vi "CRYAuto Save Editor.vi"() -> ()   [LabVIEW 2013]
uses:
  <vilib>/Utility/miscctls.llb/LVBoundsTypeDef.ctl
  Typedef Control/CRYAuto Save Cluster.ctl
  CRYProject/CRYProject Editor Global.vi
  CRYMainGlobal.vi
  CRYWindow/SubVI/CRYMain Sub Window Global.vi
panel:
  out "Auto save Bk":T1 {"Selector" items=["Space", "Underscores", "None"]}
  in  "CurLibChange":bool caption="Add Lib"
  out "EndFlag":bool
  in  "AddStep":bool
  out "Data Names":string[](array[string])
  in  "Board Tab":enum32{"Page 1"}(tab)
  in  "Cancel":bool caption="Apply"
  in  "OK":bool caption="Apply"
  in  "Main Tab":enum32{"Setting", "Help"}(tab)
  in  "Save Op":u16(slide)
  out "Control Mask3 2":bool
  out "Control Mask3":bool
  in  "DBPath":path caption="Select UDL or DSN"
  out "Control Mask2":bool
  out "Control Mask1":bool
  in  "Format Value":bool
  in  "Excel Path":path
  in  "Selector":i32(ring) caption="选择" items=["空格", "下划线", "无"]
  in  "Axes String":string
  in  "User Default":bool caption="使用默认值"
  in  "Custom header":string
  in  "Delimiter":i32(ring) caption="分隔符" items=["制表符", "逗号", "空格", "其他"]
  in  "Autosave Folder Path:":path caption="自动保存文件夹路径"
  out "Save":bool caption="保存"
  in  "Data List":i32[](listbox) caption="数据"
  out "Format":bool caption="格式"
  out "Test Information":bool caption="测试信息"
  in  "Format Op":u16(slide)
  in  "Header Op":u16(slide)
  in  "Add":bool
  in  "Clear":bool
  in  "Template":string caption="模板"
  in  "User defined":string caption="用户定义"
  in  "Operator":bool caption="操作员"
  out "Filename":bool caption="文件名称"
  in  "Character":string caption="字符"
  in  "x":bool
  in  "y":bool
  in  "z":bool
  out "Header":bool caption="标题"
  in  "Layout Op":u16(slide)
  out "Layout":bool caption="布局"
  out "Notation":bool caption="符号"
  in  "Notation Op":u16(slide)
  in  "Notation Decimal":i32 caption="位小数"
  in  "Time":bool caption="时间"
  in  "Lot No.":bool caption="批次"
  in  "Serial No.":bool caption="序号"
  in  "Prompt for comment":bool caption="注释提示"
  in  "File Name Mode1":u16(slide)
  in  "filename constr":i32(listbox)=-1 caption="构造"
  in  "File Name Mode2":u16(slide)
  in  "Axis":u16(slide) caption="轴" scale=0.0..2.0
  in  "Value":u16(ring) caption="曲线库值" items=["Max FSD Out Stimulus", "采集延迟 [Direct In 1]", "unity cal-in sens-in", "CRY33x Mic 1 sens-in", "CRY33x Mic 2 sens-in", "CRY33x Mic 3 sens-in", "CRY33x Mic 4 sens-in", "USB In L sens-in", "USB In R sens-in", "unity cal-out sens-out", "CRY602 Mouth 1 sens-out", "CRY602 Mouth 2 sens-out", "USB Out R sens-out", "Max FSD In [Direct In 1]"]
  out "single val":string
  in  "Help":string
  in  "Apply":bool
  in  "Load...":bool caption="Apply"
  in  "Save As...":bool caption="Apply"
  in  "Revert":bool caption="Apply"
  in  "fn construction":i32[](array[numeric])
  in  "Hardware In":string
  in  "Calibration In":string
  in  "Channel":i32=1
  out "Set up Out":string
  in  "Set up In":string
  in  "stop":bool
  in  "Load Test":bool=TRUE
  out "Auto save":T1 {"Selector" items=["Space", "Underscores", "None"]}
  out "VIMiniumBound":T2
  in  "Proper VI No":i32
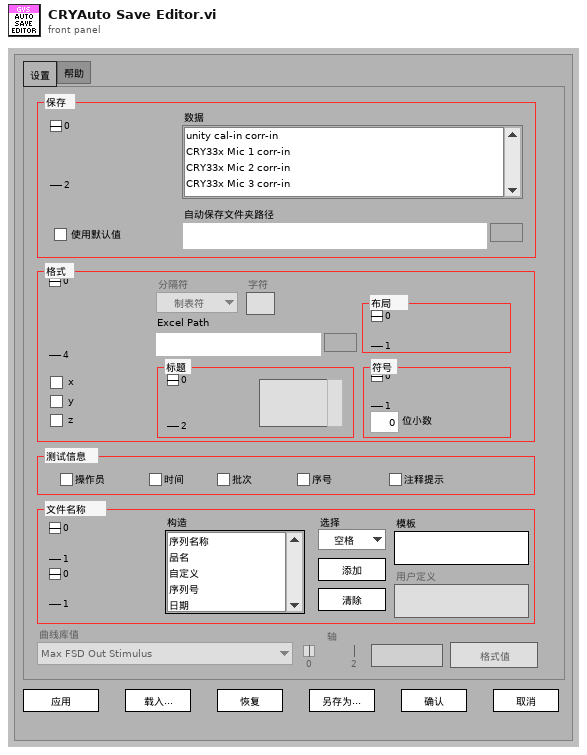
[diagram p1: front panel]
types:
  T1 = typedef "CRYAuto Save Cluster.ctl" = cluster{"Name":string, "save":enum16{"Data", "Results", "Waveforms"}, "Item Names":string[], "Autosave folder":path, "data format":u16, "filename option":enum16{"auto", "prompt"}, "fn construction":i32[], "layout":enum16{"rows", "columns"}, "notation":enum16{"sci", "float"}, "precision":i32, "prompt comment":bool, "header":enum16{"none", "standard", "custom"}, "custom header":string, "serial no.":bool, "User defined":string, "delimiter":enum16{"tab", "comma", "space", "other"}, "other delim":string, "axes":cluster{"x":bool, "y":bool, "z":bool}, "Time Stamp":bool, "Lot No.":bool, "Operator":bool, "Excel Template":string, "New or Append":u16, "Data":u16, "Help":string, "Tab Value":enum32{"Setting", "Help"}, "UDL or DSN":path, "User Default":bool, "Selector":i32, "Axis":u16, "Value Name":string, "format string":cluster{"dB Format String out":string, "Lin Format String out":string}, "DBPath":path}
  T2 = typedef "LVBoundsTypeDef.ctl" = cluster{"Width":u32, "Height":u32}
  T3 = enum32{"existing file", "new file", "new or existing file", "existing dir", "new dir", "new or existing dir", "existing file (use LLBs)", "new file (use LLBs)", "new or existing file (use LLBs)", "new or existing file or directory (use LLBs)", "existing dir (use LLBs)", "new dir (use LLBs)", "new or existing dir (use LLBs)", "existing file or dir", "new file or dir", "new or existing file or dir", "existing file or dir (use LLBs)", "new file or dir (use LLBs)"}
  T4 = typedef "CRYStep.ctl" = cluster{"No.VI":i32, "Category":string, "StepName":string, "Seq setup flattened":string, "Comment":string, "Steps config.":bool[], "Jump config":i32[], "Start":dbl, "Increment":dbl, "Name":string, "Unit":string, "Y data":u16, "Y prefix":string, "Y dB ref":dbl, "Y unit":string, "Repeat State Array":cluster{"Start":dbl, "Increment":dbl, "Count":i32, "Num":i32}[]}
  T5 = enum8{"Enabled", "Disabled", "Disabled and Grayed Out"}
  T6 = enum32{"English", "Chinese", "Korean", "Japanese", "Russian", "Chinese traditional"}
  T7 = enum16{"OK", "Yes", "YesNo", "YesNoCancel", "ReplaceAppend"}
  T8 = typedef "CRYData Cluster Array.ctl" = T9[]
  T9 = typedef "CRYData Cluster.ctl" = cluster{"Name":string, "Curve":cluster{"x":dbl, "y":dbl, "z":dbl}[], "X data":u16, "Y data":u16, "Z data":u16, "X axis":u16, "Y axis":u16, "Z axis":u16, "X unit":string, "Y unit":string, "Z unit":string, "X dB ref":dbl, "Y dB ref":dbl, "Z dB ref":dbl, "single val":bool, "protected":bool, "display X":bool, "display Y":bool, "display Z":bool, "Test Info":string, "Step No.":i32, "Plot Settings":cluster{"Color":u32, "Interpolation":u8, "Point Style":u8, "Line Style":u8, "Point Color":u32, "Line Width":u8, "Bar Plot Style":u8, "Fill To":i16}, "AutoProtect":bool}
  T10 = typedef "CRYResult Cluster Array.ctl" = T11[]
  T11 = typedef "CRYResult Cluster.ctl" = cluster{"Name":string, "Margin":dbl, "unit":string, "Verdict":bool, "Limit":string, "Max/Min":string, "protected":bool, "Step No.":i32, "Test Info":string, "AutoProtect":bool}
  T12 = typedef "CRYWaveform Cluster Array.ctl" = T13[]
  T13 = typedef "CRYWaveform Cluster.ctl" = cluster{"Waveform":cluster{"X0":dbl, "dX":dbl, "Y":sgl[]}, "X data":u16, "Y data":u16, "Y axis":u16, "X unit":string, "Y unit":string, "Y dB ref":dbl, "display Y":bool, "display X":bool, "Overload?":bool, "Test Info":string, "Step No.":i32, "Name":string, "protected":bool, "Sqc history":string[], "Signal Channel ID":i32, "Plot Settings":cluster{"Color":u32, "Interpolation":u8, "Point Style":u8, "Line Style":u8, "Point Color":u32, "Line Width":u8, "Bar Plot Style":u8, "Fill To":i16}, "AutoProtect":bool}
  T14 = cluster{"Apply":bool, "Load Test":bool, "OK":bool, "Cancel":bool}
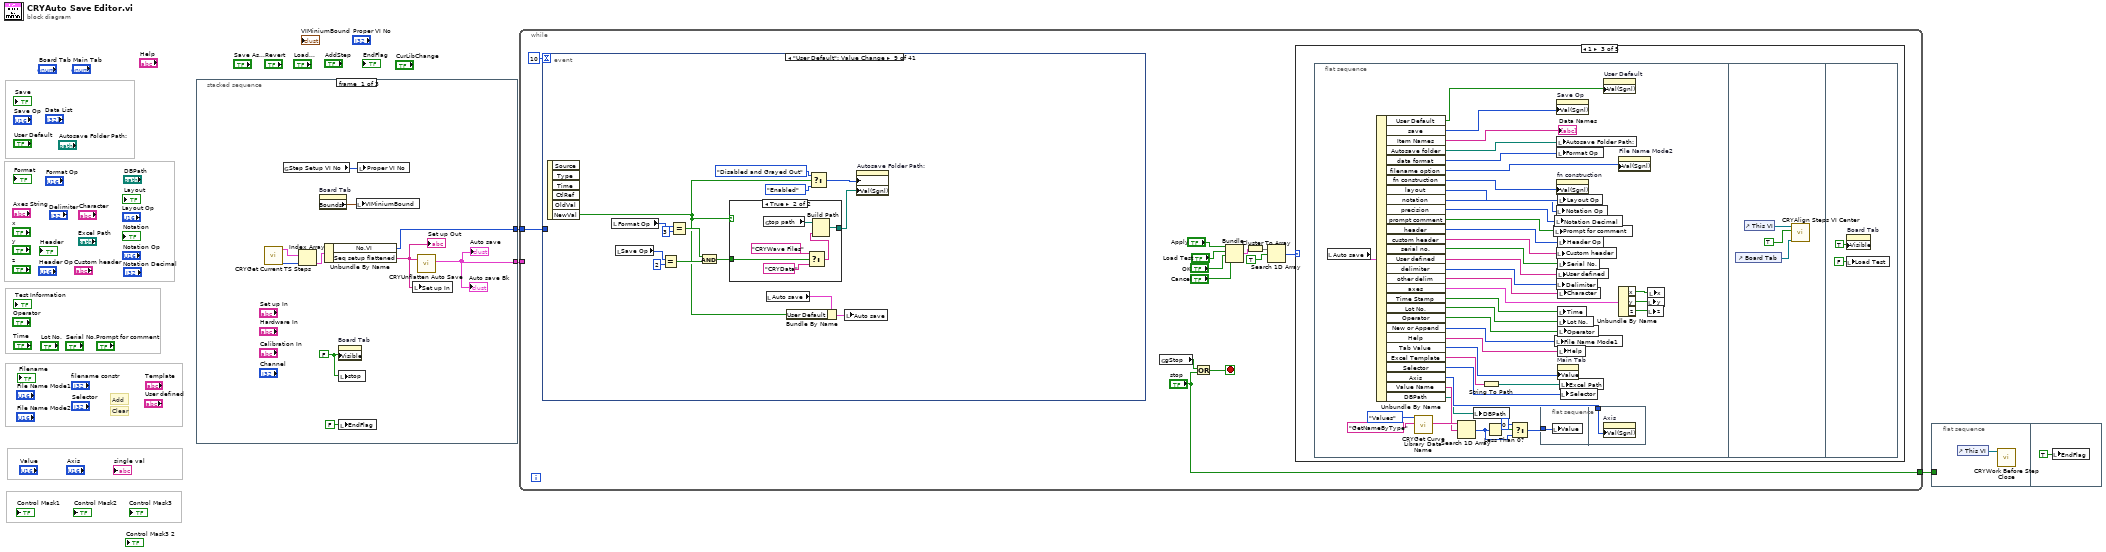
[diagram p0: block diagram]
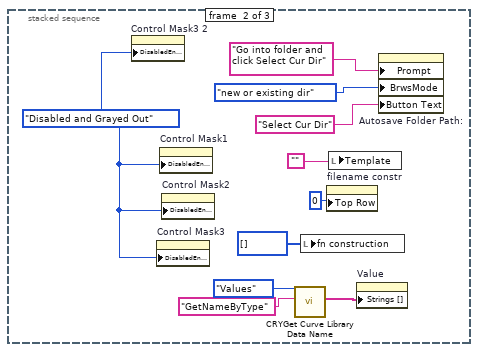
[diagram p2: hidden frame]
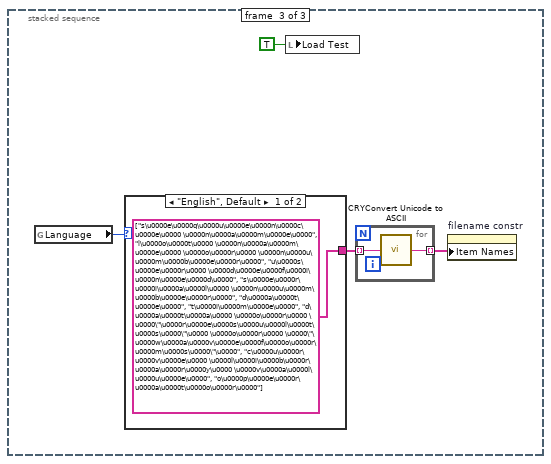
[diagram p3: hidden frame]
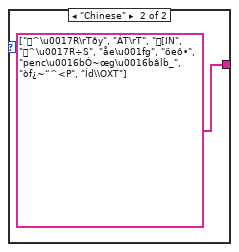
[diagram p4: hidden frame]
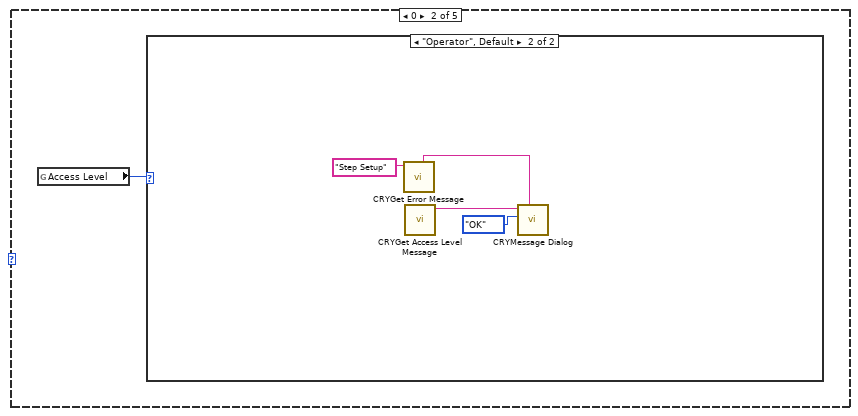
[diagram p6: hidden frame]
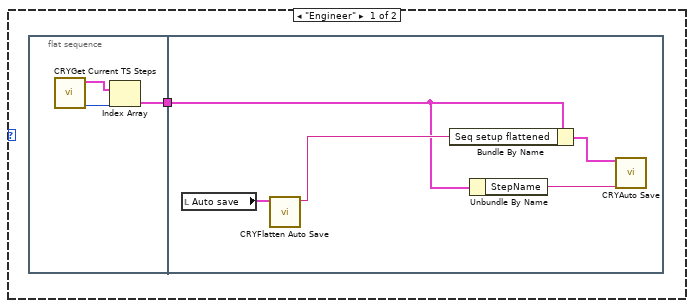
[diagram p7: hidden frame]
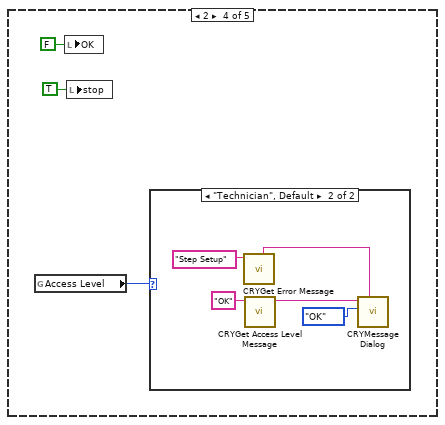
[diagram p8: hidden frame]
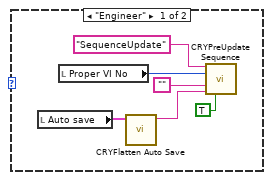
[diagram p9: hidden frame]
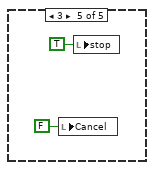
[diagram p10: hidden frame]
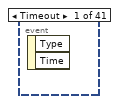
[diagram p11: hidden frame]
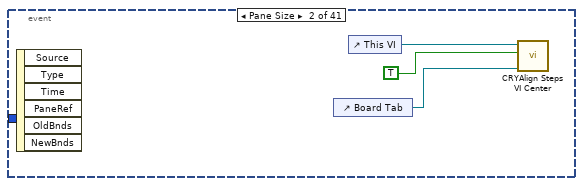
[diagram p12: hidden frame]
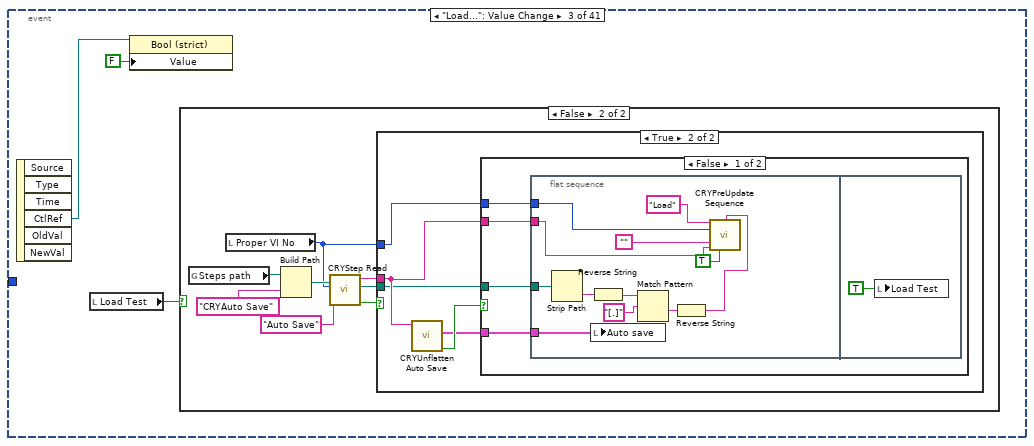
[diagram p13: hidden frame]
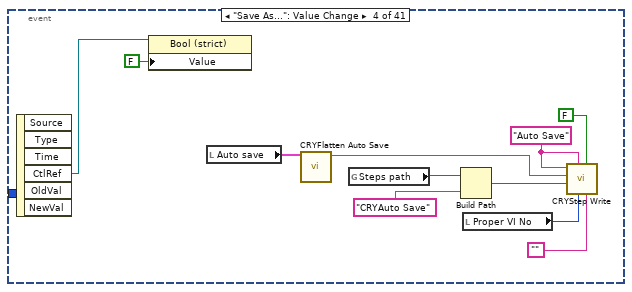
[diagram p17: hidden frame]
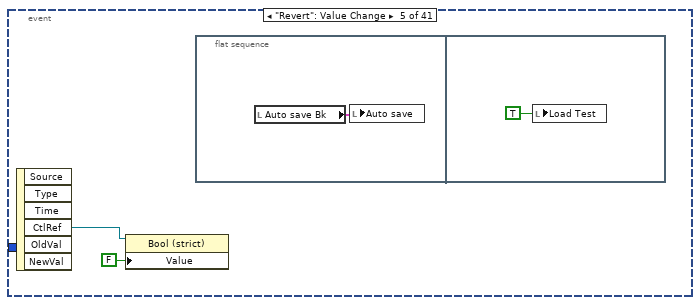
[diagram p18: hidden frame]
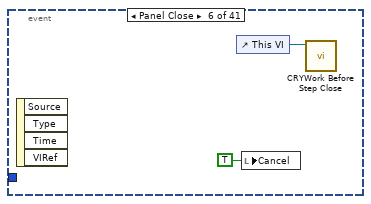
[diagram p19: hidden frame]
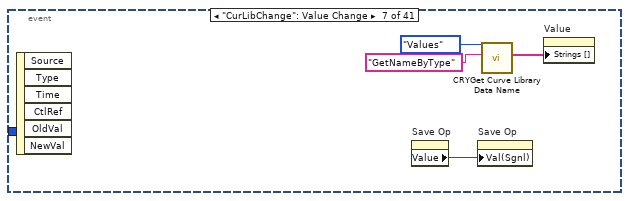
[diagram p20: hidden frame]
diagram:
  # "Clear"
  # "Add"
  n1 = stacked-sequence {
    tunnel: [w5 _ _] -> w3
    tunnel: [w6 _ _] -> w1
    frame #0 {
      w4 = FALSE ("Visible")
      n2 = call "CRYGet Current TS Steps.vi"() -> ("SelectStepNumber in Tree"=w9:i32, "Steps"=w10:T4[])  [unwired: 7 in, 3 out]
      n3 = global read "CRYProject Editor Global.vi" "Step Setup VI No"() -> (w13:i32)
      n4 = Index Array(array=w10, index=w9) -> (element=w12:T4)
      n5 = property on="Board Tab" class="TabCtl (strict)"() -> ("Bounds"=w8:T2)  [unwired: 2 in, 2 out]
      n6 = Unbundle By Name(w12) -> ("No.VI"=w6:i32, "Seq setup flattened"=w11:string)
      "Set up Out" <- w11
      n7 = property on="Board Tab" class="TabCtl (strict)"("Visible"=w4) -> ()  [unwired: 2 in, 2 out]
      n8 = local write "stop"(w4) -> ()
      n9 = local write "EndFlag"(FALSE ("EndFlag")) -> ()
      n10 = local write "VIMiniumBound"(w8) -> ()
      n11 = local write "Proper VI No"(w13) -> ()
      n12 = local write "Set up In"(w11) -> ()
      n13 = call "CRYUnflatten Auto Save.vi"("Flatten Auto Save"=w11) -> ("Auto save"=w5:T1)  [unwired: 8 in, 2 out]
      "Auto save" <- w5
      "Auto save Bk" <- w5
    }
    frame #1 {
      w14 = T5."Disabled and Grayed Out" ("Disabled")
      n14 = property on="Control Mask3 2" class="Bool (strict)"("DisabledEnum"=w14) -> ()  [unwired: 2 in, 2 out]
      n15 = property on="Control Mask3" class="Bool (strict)"("DisabledEnum"=w14) -> ()  [unwired: 2 in, 2 out]
      n16 = property on="Control Mask1" class="Bool (strict)"("DisabledEnum"=w14) -> ()  [unwired: 2 in, 2 out]
      n17 = property on="Control Mask2" class="Bool (strict)"("DisabledEnum"=w14) -> ()  [unwired: 2 in, 2 out]
      n18 = call "CRYGet Curve Library Data Name.vi"("sAction"="GetNameByType", "Type"=enum16{"Curves", "Values", "Results", "WFM"}."Values") -> ("sNames"=w16:string[])  [unwired: 6 in, 3 out]
      n19 = local write "fn construction"(i32[] [] ("fn construction")) -> ()
      n20 = property on="filename constr" class="LstBox (strict)"("Top Row"=0 ("filename constr")) -> ()  [unwired: 2 in, 2 out]
      n21 = local write "Template"("") -> ()
      n22 = property on="Value" class="Ring (strict)"("Strings []"=w16) -> ()  [unwired: 2 in, 2 out]
      n23 = property on="Autosave Folder Path:" class="Path"("Prompt"="Go into folder and click Select Cur Dir" ("prompt"), "BrwsMode"=T3."new or existing dir" ("Browse Options:Selection Mode"), "Button Text"="Select Cur Dir" ("Browse Options:Button Text")) -> ()  [unwired: 2 in, 2 out]
    }
    frame #2 {
      n24 = global read "CRYMainGlobal.vi" "Language"() -> (w26:T6)
      n25 = case shown="\"English\", Default" w26 {
        tunnel: [string[] ["s\u0000e\u0000q\u0000u\u0000e\u0000n\u0000c\u0000e\u0000 \u0000n\u0000a\u0000m\u0000e\u0000", "l\u0000o\u0000t\u0000 \u0000n\u0000a\u0000m\u0000e\u0000 \u0000o\u0000r\u0000 \u0000n\u0000u\u0000m\u0000b\u0000e\u0000r\u0000", "u\u0000s\u0000e\u0000r\u0000 \u0000d\u0000e\u0000f\u0000i\u0000n\u0000e\u0000d\u0000", "s\u0000e\u0000r\u0000i\u0000a\u0000l\u0000 \u0000n\u0000u\u0000m\u0000b\u0000e\u0000r\u0000", "d\u0000a\u0000t\u0000e\u0000", "t\u0000i\u0000m\u0000e\u0000", "d\u0000a\u0000t\u0000a\u0000 \u0000o\u0000r\u0000 \u0000\"\u0000r\u0000e\u0000s\u0000u\u0000l\u0000t\u0000s\u0000\"\u0000 \u0000o\u0000r\u0000 \u0000\"\u0000w\u0000a\u0000v\u0000e\u0000f\u0000o\u0000r\u0000m\u0000s\u0000\"\u0000", "c\u0000u\u0000r\u0000v\u0000e\u0000 \u0000l\u0000i\u0000b\u0000r\u0000a\u0000r\u0000y\u0000 \u0000v\u0000a\u0000l\u0000u\u0000e\u0000", "o\u0000p\u0000e\u0000r\u0000a\u0000t\u0000o\u0000r\u0000"] string[] ["^\u0017R\rTðy", "ÁT\rT", "ꁚ[IN", "^\u0017R÷S", "åe\u001fg", "öeô•", "penc\u0016bÓ~œg\u0016bâlb_", "òf¿~“^<P", "Íd\\OXT"]] -> w25
        frame "English", Default {
        }
        frame "Chinese" {
        }
      }
      n26 = local write "Load Test"(TRUE ("Load Test")) -> ()
      n27 = for {
        tunnel: [w31] -> w24 mode=indexing
        tunnel: w25 -> [w30] mode=indexing
        n28 = call "CRYConvert Unicode to ASCII.vi"("Unicode"=w30) -> ("ASCII"=w31:string)  [unwired: 4 in]
      }
      n29 = property on="filename constr" class="LstBox (strict)"("Item Names"=w24) -> ()  [unwired: 2 in, 2 out]
    }
  }
  n30 = while {
    tunnel: w3 -> [_]
    tunnel: ["stop"] -> w2
    tunnel: w1 -> [w35]
    stop <- w38 stop-if-true
    n31 = event shown="[8] \"User Default\": Value Change" {
      selector: _ -> [_ _ _ _ _ _ _ _ _ _ _ _ _ _ _ _ _ _ _ _ _ _ _ _ _ _ _ _ _ _ _ _ _ _ _ _ _ _ _ _ _]
      dyn-events: _ -> [_ _ _ _ _ _ _ _ _ _ _ _ _ _ _ _ _ _ _ _ _ _ _ _ _ _ _ _ _ _ _ _ _ _ _ _ _ _ _ _ _]
      timeout: 10 -> [_ _ _ _ _ _ _ _ _ _ _ _ _ _ _ _ _ _ _ _ _ _ _ _ _ _ _ _ _ _ _ _ _ _ _ _ _ _ _ _ _]
      tunnel: w35 -> [_ _ _ _ _ _ _ w183 _ _ _ _ _ _ _ _ _ _ _ _ _ _ _ _ _ _ _ _ _ _ _ _ _ _ _ _ _ _ _ _ _]
      event Timeout {
        n32 = event-data() -> ()  [unwired: 3 out]
      }
      event Pane Size {
        n33 = event-data() -> ()  [unwired: 7 out]
        n34 = control-ref of="Board Tab"() -> (w124:refnum<vi>)
        n35 = control-ref of="This VI"() -> (w123:refnum<vi>)
        n36 = call "CRYAlign Steps VI Center.vi"("Tab2"=w124, "Input/Output"=TRUE ("Preview"), "VIRef"=w123) -> ()  [unwired: 1 in, 8 out]
      }
      event "Load...": Value Change {
        n37 = event-data() -> ("CtlRef"=w126:refnum<vi>)  [unwired: 6 out]
        n38 = local read "Load Test"() -> (w128:bool)
        n39 = property class="Bool (strict)"(reference=w126, "Value"=FALSE) -> ()  [unwired: 1 in, 2 out]
        n40 = case shown="False" w128 {
          frame True {
          }
          frame False {
            n41 = global read "CRYMainGlobal.vi" "Steps path"() -> (w135:path)
            n42 = local read "Proper VI No"() -> (w130:i32)
            n43 = Build Path(base path=w135, name or relative path="CRYAuto Save") -> (appended path=w134:path)
            n44 = call "CRYStep Read.vi"("Category Name"="Auto Save", "Proper VI No"=w130, "Step File Path"=w134) -> ("status"=w132:bool, "selected path"=w129:path, "Flatten Step"=w131:string)  [unwired: 1 in, 3 out]
            n45 = case shown="True" w132 {
              tunnel: w131 -> [_ w138]
              tunnel: w130 -> [_ w139]
              tunnel: w129 -> [_ w137]
              frame False {
              }
              frame True {
                n46 = call "CRYUnflatten Auto Save.vi"("Flatten Auto Save"=w138) -> ("Error?"=w141:bool, "Auto save"=w140:T1)  [unwired: 8 in, 1 out]
                n47 = case shown="False" w141 {
                  tunnel: w140 -> [w145 _]
                  tunnel: w139 -> [w144 _]
                  tunnel: w138 -> [w143 _]
                  tunnel: w137 -> [w142 _]
                  frame False {
                    n48 = flat-sequence {
                      tunnel: w145 -> [w157]
                      tunnel: w144 -> [w154]
                      tunnel: w143 -> [w153]
                      tunnel: w142 -> [w152]
                      frame #0 {
                        n49 = Strip Path(path=w152) -> (name=w147:string)  [unwired: 1 out]
                        n50 = local write "Auto save"(w157) -> ()
                        n51 = Reverse String(1:w147) -> (0:w149:string)
                        n52 = Match Pattern(string=w149, regular expression="[.]") -> (after substring=w150:string)  [unwired: 4 out]
                        n53 = Reverse String(1:w150) -> (0:w146:string)
                        n54 = call "CRYPreUpdate Sequence.vi"("EventName"="Load", "StepName Arg3"=w146, "Proper VI No"=w154, "Project View Step Name Identifier Arg1"="", "Step flattened Arg2"=w153, "AllChangeFlg"=TRUE ("Name/Identifier")) -> ()  [unwired: 10 in]
                      }
                      frame #1 {
                        n55 = local write "Load Test"(TRUE ("Load Test")) -> ()
                      }
                    }
                  }
                  frame True {
                  }
                }
              }
            }
          }
        }
      }
      event "Save As...": Value Change {
        w163 = "Auto Save" ("Step File Name")
        n56 = event-data() -> ("CtlRef"=w159:refnum<vi>)  [unwired: 6 out]
        n57 = property class="Bool (strict)"(reference=w159, "Value"=FALSE) -> ()  [unwired: 1 in, 2 out]
        n58 = local read "Auto save"() -> (w161:T1)
        n59 = call "CRYFlatten Auto Save.vi"("Auto Save"=w161) -> ("Auto Save flattened"=w162:string)  [unwired: 10 in]
        n60 = global read "CRYMainGlobal.vi" "Steps path"() -> (w165:path)
        n61 = Build Path(base path=w165, name or relative path="CRYAuto Save") -> (appended path=w164:path)
        n62 = local read "Proper VI No"() -> (w168:i32)
        n63 = call "CRYStep Write.vi"("StepIdentifier"="", "Default"=FALSE, "Proper VI No"=w168, "Category Name"=w163, "Step File Path"=w164, "Step flattened"=w162, "Step File Name"=w163) -> ()  [unwired: 1 in, 4 out]
      }
      event "Revert": Value Change {
        n64 = event-data() -> ("CtlRef"=w171:refnum<vi>)  [unwired: 6 out]
        n65 = property class="Bool (strict)"(reference=w171, "Value"=FALSE) -> ()  [unwired: 1 in, 2 out]
        n66 = flat-sequence {
          frame #0 {
            n67 = local read "Auto save Bk"() -> (w172:T1)
            n68 = local write "Auto save"(w172) -> ()
          }
          frame #1 {
            n69 = local write "Load Test"(TRUE ("Load Test")) -> ()
          }
        }
      }
      event Panel Close {
        n70 = event-data() -> ()  [unwired: 5 out]
        n71 = control-ref of="This VI"() -> (w175:refnum<vi>)
        n72 = local write "Cancel"(TRUE ("Cancel")) -> ()
        n73 = call "CRYWork Before Step Close.vi"("StepVI Ref"=w175) -> ()  [unwired: 11 in]
      }
      event "CurLibChange": Value Change {
        n74 = event-data() -> ()  [unwired: 7 out]
        n75 = property on="Save Op" class="Slide (strict)"() -> ("Value"=w176:u16)  [unwired: 2 in, 2 out]
        n76 = property on="Save Op" class="Slide (strict)"("Val(Sgnl)"=w176) -> ()  [unwired: 2 in, 2 out]
        n77 = call "CRYGet Curve Library Data Name.vi"("sAction"="GetNameByType", "Type"=enum16{"Curves", "Values", "Results", "WFM"}."Values") -> ("sNames"=w179:string[])  [unwired: 6 in, 3 out]
        n78 = property on="Value" class="Ring (strict)"("Strings []"=w179) -> ()  [unwired: 2 in, 2 out]
      }
      event "Save Op": Value Change {
        n79 = event-data() -> ("NewVal"=w189:u16)  [unwired: 6 out]
        n80 = global read "CRYMainGlobal.vi" "On/Off Line"() -> (w187:bool)
        n81 = call "CRYGet Error Message.vi"("Kind"="Auto Save Sub") -> ("Unicode Message Sub"=w185:string[])  [unwired: 5 in, 5 out]
        n82 = for {
          tunnel: w185 -> [w197] mode=indexing
          tunnel: [w196] -> w184 mode=indexing
          n83 = call "CRYConvert Unicode to ASCII.vi"("Unicode"=w197) -> ("ASCII"=w196:string)  [unwired: 4 in]
        }
        n84 = Index Array(array=w184, index=w189) -> (element=w188:string)
        n85 = case shown="2" w189 {
          tunnel: w183 -> [w206 w231 w246]
          tunnel: [w205 w230 w245] -> w193
          tunnel: [enum16{"Data", "Results", "Waveforms"}."Data" ("save") enum16{"Data", "Results", "Waveforms"}."Results" ("save") enum16{"Data", "Results", "Waveforms"}."Waveforms" ("save")] -> w191
          tunnel: w188 -> [w203 w228 w243]
          tunnel: w187 -> [w202 w227 w242]
          tunnel: [w201 w226 w241] -> w182
          frame 0, Default {
            n86 = case shown="True" w202 {
              tunnel: enum16{"Curves", "Values", "Results", "WFM"}."Curves" ("Type In") -> [w215 w221]
              tunnel: enum16{"Curves", "Values", "Results", "WFM"}."Values" ("Type In") -> [w216 w220]
              tunnel: [w214 w219] -> w210
              tunnel: [w213 w218] -> w209
              tunnel: w206 -> [_ w217]
              frame False {
                n87 = call "CRYGet Curve Library Array.vi"("Type In"=w215) -> ("Curve/Value array"=w214:T8)  [unwired: 10 out]
                n88 = call "CRYGet Curve Library Array.vi"("Type In"=w216) -> ("Curve/Value array"=w213:T8)  [unwired: 10 out]
              }
              frame True {
                n89 = call "CRYGet Upper Step Data.vi"("Type In"=w221, "No.VI"=w217) -> ("Curve array"=w219:T8)  [unwired: 9 out]
                n90 = call "CRYGet Upper Step Data.vi"("Type In"=w220, "No.VI"=w217) -> ("Value array"=w218:T8)  [unwired: 9 out]
              }
            }
            n91 = for {
              tunnel: w210 -> [w225] mode=indexing
              tunnel: [w224] -> w208 mode=indexing
              n92 = Unbundle By Name(w225) -> ("Name"=w224:string)
            }
            n93 = for {
              tunnel: w209 -> [w223] mode=indexing
              tunnel: [w222] -> w207 mode=indexing
              n94 = Unbundle By Name(w223) -> ("Name"=w222:string)
            }
            n95 = Build Array (concatenate)(w208, w207) -> (w205:string[])
            n96 = property on="Data List" class="LstBox (strict)"("Item Names"=w205, "Caption.Text"=w203) -> (error out=w201:errorcluster)  [unwired: 2 in, 1 out]
          }
          frame 1 {
            n97 = case shown="True" w227 {
              tunnel: enum16{"Curves", "Values", "Results", "WFM"}."Results" ("Type In") -> [w235 w238]
              tunnel: [w234 w237] -> w232
              tunnel: w231 -> [_ w236]
              frame False {
                n98 = call "CRYGet Curve Library Array.vi"("Type In"=w235) -> ("Result array"=w234:T10)  [unwired: 10 out]
              }
              frame True {
                n99 = call "CRYGet Upper Step Data.vi"("Type In"=w238, "No.VI"=w236) -> ("Result array"=w237:T10)  [unwired: 9 out]
              }
            }
            n100 = for {
              tunnel: w232 -> [w240] mode=indexing
              tunnel: [w239] -> w230 mode=indexing
              n101 = Unbundle By Name(w240) -> ("Name"=w239:string)
            }
            n102 = property on="Data List" class="LstBox (strict)"("Item Names"=w230, "Caption.Text"=w228) -> (error out=w226:errorcluster)  [unwired: 2 in, 1 out]
          }
          frame 2 {
            n103 = case shown="True" w242 {
              tunnel: enum16{"Curves", "Values", "Results", "WFM"}."WFM" ("Type In") -> [w250 w253]
              tunnel: [w249 w252] -> w247
              tunnel: w246 -> [_ w251]
              frame False {
                n104 = call "CRYGet Curve Library Array.vi"("Type In"=w250) -> ("Waveform Array"=w249:T12)  [unwired: 10 out]
              }
              frame True {
                n105 = call "CRYGet Upper Step Data.vi"("Type In"=w253, "No.VI"=w251) -> ("Waveform Array"=w252:T12)  [unwired: 9 out]
              }
            }
            n106 = for {
              tunnel: w247 -> [w255] mode=indexing
              tunnel: [w254] -> w245 mode=indexing
              n107 = Unbundle By Name(w255) -> ("Name"=w254:string)
            }
            n108 = property on="Data List" class="LstBox (strict)"("Item Names"=w245, "Caption.Text"=w243) -> (error out=w241:errorcluster)  [unwired: 2 in, 1 out]
          }
        }
        n109 = local read "Data Names"() -> (w192:string[])
        n110 = local read "Auto save"() -> (w194:T1)
        n111 = local read "Format Op"() -> (w195:u16)
        n112 = Bundle By Name(cluster=w194, "save"=w191) -> (w186:T1)
        n113 = for {
          tunnel: w193 -> [w199]
          tunnel: w192 -> [w200] mode=indexing
          tunnel: [w198] -> w181 mode=indexing
          n114 = Search 1D Array(1D array=w199, element=w200) -> (index of element=w198:i32)  [unwired: 1 in]
        }
        n115 = property on="Data List" class="LstBox (strict)"(error in=w182, "Top Row"=0) -> ()  [unwired: 1 in, 2 out]
        n116 = local write "Auto save"(w186) -> ()
        n117 = property on="Format Op" class="Slide (strict)"("Val(Sgnl)"=w195) -> ()  [unwired: 2 in, 2 out]
        n118 = local write "Data List"(w181) -> ()
      }
      event "User Default": Value Change {
        n119 = event-data() -> ("NewVal"=w257:bool)  [unwired: 6 out]
        n120 = local read "Format Op"() -> (w264:u16)
        n121 = local read "Save Op"() -> (w261:u16)
        n122 = Equal?(x=w261, y=u16 2) -> (x = y?=w259:bool)
        n123 = Equal?(x=w264, y=u16 3) -> (x = y?=w260:bool)
        n124 = And(x=w260, y=w259) -> (x .and. y?=w258:bool)
        n125 = case shown="True" w257 {
          tunnel: [w270 w274] -> w263
          tunnel: w258 -> [_ w276]
          frame False {
            n126 = local read "Autosave Folder Path:"() -> (w270:path)
          }
          frame True {
            n127 = global read "CRYMainGlobal.vi" "top path"() -> (w275:path)
            n128 = Select(t="CRYWave Files", s=w276, f="CRYData") -> (s? t:f=w271:string)
            n129 = Build Path(base path=w275, name or relative path=w271) -> (appended path=w274:path)
          }
        }
        n130 = local read "Auto save"() -> (w269:T1)
        n131 = Bundle By Name(cluster=w269, "User Default"=w257) -> (w268:T1)
        n132 = Select(t=T5."Disabled and Grayed Out" ("Disabled"), s=w257, f=T5."Enabled" ("Disabled")) -> (s? t:f=w256:T5)
        n133 = local write "Auto save"(w268) -> ()
        n134 = property on="Autosave Folder Path:" class="Path"("DisabledEnum"=w256, "Val(Sgnl)"=w263) -> ()  [unwired: 2 in, 2 out]
      }
      event "Format Op": Value Change {
        n135 = event-data() -> ("NewVal"=w278:u16)  [unwired: 6 out]
        n136 = case shown="4" w278 {
          frame 0, Default {
            w281 = TRUE ("Visible")
            w280 = FALSE ("Visible")
            w283 = T5."Enabled" ("Disabled")
            # "Text"
            n137 = property on="x" class="Bool (strict)"("DisabledEnum"=w283) -> ()  [unwired: 2 in, 2 out]
            n138 = property on="Delimiter" class="Ring (strict)"("DisabledEnum"=w283) -> ()  [unwired: 2 in, 2 out]
            n139 = property on="Notation Decimal" class="DigNum (strict)"("DisabledEnum"=w283) -> ()  [unwired: 2 in, 2 out]
            n140 = property on="Operator" class="Bool (strict)"("DisabledEnum"=w283) -> ()  [unwired: 2 in, 2 out]
            n141 = property on="Prompt for comment" class="Bool (strict)"("DisabledEnum"=w283) -> ()  [unwired: 2 in, 2 out]
            n142 = property on="Excel Path" class="Path"("DisabledEnum"=T5."Disabled and Grayed Out" ("Disabled")) -> ()  [unwired: 2 in, 2 out]
            n143 = property on="y" class="Bool (strict)"("DisabledEnum"=w283) -> ()  [unwired: 2 in, 2 out]
            n144 = property on="Layout Op" class="Slide (strict)"("DisabledEnum"=w283) -> ()  [unwired: 2 in, 2 out]
            n145 = property on="Time" class="Bool (strict)"("DisabledEnum"=w283) -> ()  [unwired: 2 in, 2 out]
            n146 = property on="Header Op" class="Slide (strict)"("DisabledEnum"=w283) -> ()  [unwired: 2 in, 2 out]
            n147 = property on="z" class="Bool (strict)"("DisabledEnum"=w283) -> ()  [unwired: 2 in, 2 out]
            n148 = property on="Notation Op" class="Slide (strict)"("DisabledEnum"=w283) -> ()  [unwired: 2 in, 2 out]
            n149 = property on="Lot No." class="Bool (strict)"("DisabledEnum"=w283) -> ()  [unwired: 2 in, 2 out]
            n150 = property on="Serial No." class="Bool (strict)"("DisabledEnum"=w283) -> ()  [unwired: 2 in, 2 out]
            n151 = local read "Header Op"() -> (w284:u16)
            n152 = local read "Delimiter"() -> (w285:i32)
            n153 = property on="Delimiter" class="Ring (strict)"("Val(Sgnl)"=w285) -> ()  [unwired: 2 in, 2 out]
            n154 = property on="Header Op" class="Slide (strict)"("Val(Sgnl)"=w284) -> ()  [unwired: 2 in, 2 out]
            n155 = property on="Control Mask1" class="Bool (strict)"("Visible"=w280) -> ()  [unwired: 2 in, 2 out]
            n156 = property on="Control Mask2" class="Bool (strict)"("Visible"=w280) -> ()  [unwired: 2 in, 2 out]
            n157 = property on="DBPath" class="Path"("Visible"=w280) -> ()  [unwired: 2 in, 2 out]
            n158 = property on="Control Mask3" class="Bool (strict)"("Visible"=w280) -> ()  [unwired: 2 in, 2 out]
            n159 = property on="Layout" class="Bool (strict)"("Visible"=w281) -> ()  [unwired: 2 in, 2 out]
            n160 = property on="Layout Op" class="Slide (strict)"("Visible"=w281) -> ()  [unwired: 2 in, 2 out]
          }
          frame 1 {
            w287 = TRUE ("Visible")
            w286 = FALSE ("Visible")
            w289 = T5."Enabled" ("Disabled")
            w288 = T5."Disabled and Grayed Out" ("Disabled")
            # "DAT/RES/WFM"
            # "Result"
            n161 = property on="Operator" class="Bool (strict)"("DisabledEnum"=w289) -> ()  [unwired: 2 in, 2 out]
            n162 = property on="Prompt for comment" class="Bool (strict)"("DisabledEnum"=w289) -> ()  [unwired: 2 in, 2 out]
            n163 = property on="Time" class="Bool (strict)"("DisabledEnum"=w289) -> ()  [unwired: 2 in, 2 out]
            n164 = property on="x" class="Bool (strict)"("DisabledEnum"=w288) -> ()  [unwired: 2 in, 2 out]
            n165 = property on="Delimiter" class="Ring (strict)"("DisabledEnum"=w288) -> ()  [unwired: 2 in, 2 out]
            n166 = property on="Notation Decimal" class="DigNum (strict)"("DisabledEnum"=w288) -> ()  [unwired: 2 in, 2 out]
            n167 = property on="Lot No." class="Bool (strict)"("DisabledEnum"=w289) -> ()  [unwired: 2 in, 2 out]
            n168 = property on="y" class="Bool (strict)"("DisabledEnum"=w288) -> ()  [unwired: 2 in, 2 out]
            n169 = property on="Layout Op" class="Slide (strict)"("DisabledEnum"=w288) -> ()  [unwired: 2 in, 2 out]
            n170 = property on="Header Op" class="Slide (strict)"("DisabledEnum"=w288) -> ()  [unwired: 2 in, 2 out]
            n171 = property on="Serial No." class="Bool (strict)"("DisabledEnum"=w289) -> ()  [unwired: 2 in, 2 out]
            n172 = property on="z" class="Bool (strict)"("DisabledEnum"=w288) -> ()  [unwired: 2 in, 2 out]
            n173 = property on="Notation Op" class="Slide (strict)"("DisabledEnum"=w288) -> ()  [unwired: 2 in, 2 out]
            n174 = property on="Custom header" class="Str"("DisabledEnum"=w288) -> ()  [unwired: 2 in, 2 out]
            n175 = property on="Excel Path" class="Path"("DisabledEnum"=w288) -> ()  [unwired: 2 in, 2 out]
            n176 = property on="Control Mask1" class="Bool (strict)"("Visible"=w286) -> ()  [unwired: 2 in, 2 out]
            n177 = property on="Control Mask2" class="Bool (strict)"("Visible"=w286) -> ()  [unwired: 2 in, 2 out]
            n178 = property on="Control Mask3" class="Bool (strict)"("Visible"=w286) -> ()  [unwired: 2 in, 2 out]
            n179 = property on="DBPath" class="Path"("Visible"=w286) -> ()  [unwired: 2 in, 2 out]
            n180 = property on="Layout" class="Bool (strict)"("Visible"=w287) -> ()  [unwired: 2 in, 2 out]
            n181 = property on="Layout Op" class="Slide (strict)"("Visible"=w287) -> ()  [unwired: 2 in, 2 out]
          }
          frame 2 {
            w291 = TRUE ("Visible")
            w290 = FALSE ("Visible")
            # "Excel"
            n182 = local read "Save Op"() -> (w292:u16)
            n183 = Equal?(x=w292, y=u16 2) -> (x = y?=w294:bool)
            n184 = case shown="False" w294 {
              frame False {
                w295 = T5."Enabled" ("Disabled")
                n185 = property on="x" class="Bool (strict)"("DisabledEnum"=w295) -> ()  [unwired: 2 in, 2 out]
                n186 = property on="Layout Op" class="Slide (strict)"("DisabledEnum"=w295) -> ()  [unwired: 2 in, 2 out]
                n187 = property on="Notation Decimal" class="DigNum (strict)"("DisabledEnum"=w295) -> ()  [unwired: 2 in, 2 out]
                n188 = property on="Operator" class="Bool (strict)"("DisabledEnum"=w295) -> ()  [unwired: 2 in, 2 out]
                n189 = property on="Prompt for comment" class="Bool (strict)"("DisabledEnum"=w295) -> ()  [unwired: 2 in, 2 out]
                n190 = property on="y" class="Bool (strict)"("DisabledEnum"=w295) -> ()  [unwired: 2 in, 2 out]
                n191 = property on="Time" class="Bool (strict)"("DisabledEnum"=w295) -> ()  [unwired: 2 in, 2 out]
                n192 = property on="Notation Op" class="Slide (strict)"("DisabledEnum"=w295) -> ()  [unwired: 2 in, 2 out]
                n193 = property on="Delimiter" class="Ring (strict)"("DisabledEnum"=T5."Disabled and Grayed Out" ("Disabled")) -> ()  [unwired: 2 in, 2 out]
                n194 = property on="Header Op" class="Slide (strict)"("DisabledEnum"=w295) -> ()  [unwired: 2 in, 2 out]
                n195 = property on="Excel Path" class="Path"("DisabledEnum"=w295) -> ()  [unwired: 2 in, 2 out]
                n196 = property on="z" class="Bool (strict)"("DisabledEnum"=w295) -> ()  [unwired: 2 in, 2 out]
                n197 = property on="Lot No." class="Bool (strict)"("DisabledEnum"=w295) -> ()  [unwired: 2 in, 2 out]
                n198 = property on="Serial No." class="Bool (strict)"("DisabledEnum"=w295) -> ()  [unwired: 2 in, 2 out]
                n199 = local read "Header Op"() -> (w298:u16)
                n200 = local read "Delimiter"() -> (w297:i32)
                n201 = property on="Delimiter" class="Ring (strict)"("Val(Sgnl)"=w297) -> ()  [unwired: 2 in, 2 out]
                n202 = property on="Header Op" class="Slide (strict)"("Val(Sgnl)"=w298) -> ()  [unwired: 2 in, 2 out]
              }
              frame True {
                w305 = u16 1 items=["Text", "DAT, RES, WFM", "DB", "Excel", "Wave"] ("Format Op")
                # "Wave"
                n203 = call "CRYGet Error Message.vi"("Error No"=28, "Kind"="Auto Save") -> ("Message Sub 3"=w301:string, "Window Title"=w302:string)  [unwired: 4 in, 4 out]
                n204 = call "CRYMessage Dialog.vi"("Window Title"=w302, "YesNoCancel"=T7."OK", "Message Content"=w301) -> ("YesNo"=w299:bool)  [unwired: 7 in, 1 out]
                n205 = case shown="True" w299 {
                  tunnel: w305 -> [_ w306]
                  frame False {
                  }
                  frame True {
                    n206 = property on="Format Op" class="Slide (strict)"("Val(Sgnl)"=w306) -> ()  [unwired: 2 in, 2 out]
                  }
                }
                n207 = local write "Format Op"(w305) -> ()
              }
            }
            n208 = property on="DBPath" class="Path"("Visible"=w290) -> ()  [unwired: 2 in, 2 out]
            n209 = property on="Control Mask1" class="Bool (strict)"("Visible"=w290) -> ()  [unwired: 2 in, 2 out]
            n210 = property on="Control Mask2" class="Bool (strict)"("Visible"=w290) -> ()  [unwired: 2 in, 2 out]
            n211 = property on="Control Mask3" class="Bool (strict)"("Visible"=w290) -> ()  [unwired: 2 in, 2 out]
            n212 = property on="Layout" class="Bool (strict)"("Visible"=w291) -> ()  [unwired: 2 in, 2 out]
            n213 = property on="Layout Op" class="Slide (strict)"("Visible"=w291) -> ()  [unwired: 2 in, 2 out]
          }
          frame 3 {
            w308 = TRUE ("Visible")
            w307 = FALSE ("Visible")
            # "Wave"
            n214 = local read "Save Op"() -> (w309:u16)
            n215 = case shown="0, 1" w309 {
              selector: w309 -> [_ w311]
              frame 2, Default {
                w310 = T5."Disabled and Grayed Out" ("Disabled")
                # "DATA, Wave"
                n216 = property on="x" class="Bool (strict)"("DisabledEnum"=w310) -> ()  [unwired: 2 in, 2 out]
                n217 = property on="Delimiter" class="Ring (strict)"("DisabledEnum"=w310) -> ()  [unwired: 2 in, 2 out]
                n218 = property on="Notation Decimal" class="DigNum (strict)"("DisabledEnum"=w310) -> ()  [unwired: 2 in, 2 out]
                n219 = property on="Operator" class="Bool (strict)"("DisabledEnum"=w310) -> ()  [unwired: 2 in, 2 out]
                n220 = property on="Prompt for comment" class="Bool (strict)"("DisabledEnum"=w310) -> ()  [unwired: 2 in, 2 out]
                n221 = property on="y" class="Bool (strict)"("DisabledEnum"=w310) -> ()  [unwired: 2 in, 2 out]
                n222 = property on="Layout Op" class="Slide (strict)"("DisabledEnum"=w310) -> ()  [unwired: 2 in, 2 out]
                n223 = property on="Time" class="Bool (strict)"("DisabledEnum"=w310) -> ()  [unwired: 2 in, 2 out]
                n224 = property on="Header Op" class="Slide (strict)"("DisabledEnum"=w310) -> ()  [unwired: 2 in, 2 out]
                n225 = property on="z" class="Bool (strict)"("DisabledEnum"=w310) -> ()  [unwired: 2 in, 2 out]
                n226 = property on="Serial No." class="Bool (strict)"("DisabledEnum"=w310) -> ()  [unwired: 2 in, 2 out]
                n227 = property on="Notation Op" class="Slide (strict)"("DisabledEnum"=w310) -> ()  [unwired: 2 in, 2 out]
                n228 = property on="Lot No." class="Bool (strict)"("DisabledEnum"=w310) -> ()  [unwired: 2 in, 2 out]
                n229 = property on="Custom header" class="Str"("DisabledEnum"=w310) -> ()  [unwired: 2 in, 2 out]
                n230 = property on="Excel Path" class="Path"("DisabledEnum"=w310) -> ()  [unwired: 2 in, 2 out]
              }
              frame 0, 1 {
                w317 = u16 0 items=["Text", "DAT, RES, WFM", "DB", "Excel", "Wave"] ("Format Op")
                # "Result"
                n231 = disable-structure shown="Disabled" {
                  disable-tunnel: w311 -> [w319 _]
                  frame Disabled {
                    n232 = Equal To 0?(x=w319) -> (x = 0?=w318:bool)
                    n233 = Select(s=w318) -> ()  [unwired: 2 in, 1 out]
                  }
                  frame Enabled {
                  }
                }
                n234 = call "CRYGet Error Message.vi"("Error No"=29, "Kind"="Auto Save") -> ("Message Sub 3"=w313:string, "Window Title"=w312:string)  [unwired: 4 in, 4 out]
                n235 = call "CRYMessage Dialog.vi"("Window Title"=w312, "YesNoCancel"=T7."OK", "Message Content"=w313) -> ()  [unwired: 7 in, 2 out]
                n236 = property on="Format Op" class="Slide (strict)"("Val(Sgnl)"=w317) -> ()  [unwired: 2 in, 2 out]
              }
            }
            n237 = property on="Control Mask3" class="Bool (strict)"("Visible"=w307) -> ()  [unwired: 2 in, 2 out]
            n238 = property on="DBPath" class="Path"("Visible"=w307) -> ()  [unwired: 2 in, 2 out]
            n239 = property on="Control Mask1" class="Bool (strict)"("Visible"=w307) -> ()  [unwired: 2 in, 2 out]
            n240 = property on="Control Mask2" class="Bool (strict)"("Visible"=w307) -> ()  [unwired: 2 in, 2 out]
            n241 = property on="Layout" class="Bool (strict)"("Visible"=w308) -> ()  [unwired: 2 in, 2 out]
            n242 = property on="Layout Op" class="Slide (strict)"("Visible"=w308) -> ()  [unwired: 2 in, 2 out]
          }
          frame 4 {
            n243 = local read "Save Op"() -> (w320:u16)
            n244 = Equal?(x=w320, y=u16 2) -> (x = y?=w322:bool)
            n245 = case shown="False" w322 {
              frame False {
                w323 = FALSE ("Visible")
                w324 = TRUE ("Visible")
                n246 = property on="Control Mask1" class="Bool (strict)"("Visible"=w324) -> ()  [unwired: 2 in, 2 out]
                n247 = property on="Control Mask2" class="Bool (strict)"("Visible"=w324) -> ()  [unwired: 2 in, 2 out]
                n248 = property on="DBPath" class="Path"("Visible"=w324) -> ()  [unwired: 2 in, 2 out]
                n249 = property on="Control Mask3" class="Bool (strict)"("Visible"=w324) -> ()  [unwired: 2 in, 2 out]
                n250 = property on="Layout" class="Bool (strict)"("Visible"=w323) -> ()  [unwired: 2 in, 2 out]
                n251 = property on="Layout Op" class="Slide (strict)"("Visible"=w323) -> ()  [unwired: 2 in, 2 out]
              }
              frame True {
                w331 = u16 1 items=["Text", "DAT, RES, WFM", "DB", "Excel", "Wave"] ("Format Op")
                # "Wave"
                n252 = call "CRYGet Error Message.vi"("Error No"=34, "Kind"="Auto Save") -> ("Message Sub 3"=w327:string, "Window Title"=w328:string)  [unwired: 4 in, 4 out]
                n253 = call "CRYMessage Dialog.vi"("Window Title"=w328, "YesNoCancel"=T7."OK", "Message Content"=w327) -> ("YesNo"=w325:bool)  [unwired: 7 in, 1 out]
                n254 = case shown="True" w325 {
                  tunnel: w331 -> [_ w332]
                  frame False {
                  }
                  frame True {
                    n255 = property on="Format Op" class="Slide (strict)"("Val(Sgnl)"=w332) -> ()  [unwired: 2 in, 2 out]
                  }
                }
                n256 = local write "Format Op"(w331) -> ()
              }
            }
          }
        }
        n257 = local read "Auto save"() -> (w279:T1)
        n258 = Bundle By Name(cluster=w279, "data format"=w278) -> (w277:T1)
        n259 = local write "Auto save"(w277) -> ()
      }
      event "DBPath": Value Change {
        n260 = event-data() -> ("NewVal"=w333:path)  [unwired: 6 out]
        n261 = local read "Auto save"() -> (w335:T1)
        n262 = Bundle By Name(cluster=w335, "DBPath"=w333) -> (w334:T1)
        n263 = local write "Auto save"(w334) -> ()
      }
      event "Delimiter": Value Change {
        n264 = event-data() -> ("NewVal"=w339:i32)  [unwired: 6 out]
        n265 = case shown="0..2, Default" w339 {
          tunnel: [T5."Disabled and Grayed Out" ("Disabled") T5."Enabled" ("Disabled")] -> w338
          frame 0..2, Default {
          }
          frame 3 {
          }
        }
        n266 = local read "Auto save"() -> (w337:T1)
        n267 = Bundle By Name(cluster=w337, "delimiter"=w339) -> (w336:T1)
        n268 = local write "Auto save"(w336) -> ()
        n269 = property on="Character" class="Str"("DisabledEnum"=w338) -> ()  [unwired: 2 in, 2 out]
      }
      event "Header Op": Value Change {
        n270 = event-data() -> ("NewVal"=w345:u16)  [unwired: 6 out]
        n271 = case shown="0, 1, Default" w345 {
          tunnel: [T5."Disabled and Grayed Out" ("Disabled") T5."Enabled" ("Disabled")] -> w344
          frame 0, 1, Default {
          }
          frame 2 {
          }
        }
        n272 = local read "Auto save"() -> (w343:T1)
        n273 = Bundle By Name(cluster=w343, "header"=w345) -> (w342:T1)
        n274 = local write "Auto save"(w342) -> ()
        n275 = property on="Custom header" class="Str"("DisabledEnum"=w344) -> ()  [unwired: 2 in, 2 out]
      }
      event "File Name Mode1": Value Change {
        n276 = event-data() -> ("NewVal"=w350:u16)  [unwired: 6 out]
        n277 = local read "Auto save"() -> (w349:T1)
        n278 = Bundle By Name(cluster=w349, "New or Append"=w350) -> (w348:T1)
        n279 = local write "Auto save"(w348) -> ()
      }
      event "Selector": Value Change {
        n280 = event-data() -> ("NewVal"=w351:i32)  [unwired: 6 out]
        n281 = local read "Auto save"() -> (w353:T1)
        n282 = Bundle By Name(cluster=w353, "Selector"=w351) -> (w352:T1)
        n283 = local write "Auto save"(w352) -> ()
      }
      event "Excel Path": Value Change {
        n284 = event-data() -> ("NewVal"=w355:path)  [unwired: 6 out]
        n285 = Path To String(path=w355) -> (string=w354:string)
        n286 = local read "Auto save"() -> (w357:T1)
        n287 = Bundle By Name(cluster=w357, "Excel Template"=w354) -> (w356:T1)
        n288 = local write "Auto save"(w356) -> ()
      }
      event "Add": Value Change {
        n289 = event-data() -> ()  [unwired: 7 out]
        n290 = global read "CRYMainGlobal.vi" "Language"() -> (w360:T6)
        n291 = case shown="\"Chinese\"" w360 {
          tunnel: [string[] ["<\u0000s\u0000e\u0000q\u0000>\u0000", "<\u0000l\u0000o\u0000t\u0000>\u0000", "<\u0000u\u0000s\u0000e\u0000r\u0000>\u0000", "<\u0000s\u0000n\u0000>\u0000", "<\u0000d\u0000a\u0000t\u0000e\u0000>\u0000", "<\u0000t\u0000i\u0000m\u0000e\u0000>\u0000", "<\u0000d\u0000 \u0000o\u0000r\u0000 \u0000r\u0000>\u0000", "<\u0000c\u0000l\u0000v\u0000a\u0000l\u0000>\u0000", "<\u0000o\u0000p\u0000e\u0000r\u0000>\u0000"] string[] ["<\u0000^\u0017R\rTðy>\u0000", "<\u0000ÁT\rT>\u0000", "<\u0000ꁚ[IN>\u0000", "<\u0000^\u0017R÷S>\u0000", "<\u0000åe\u001fg>\u0000", "<\u0000öeô•>\u0000", "<\u0000penc\u0016bÓ~œg\u0016bâl>\u0000", "<\u0000òf¿~“^<P>\u0000", "<\u0000Íd\\OXT>\u0000"]] -> w359
          frame "English", Default {
          }
          frame "Chinese" {
          }
        }
        n292 = for {
          tunnel: [w363] -> w358 mode=indexing
          tunnel: w359 -> [w362] mode=indexing
          n293 = call "CRYConvert Unicode to ASCII.vi"("Unicode"=w362) -> ("ASCII"=w363:string)  [unwired: 4 in]
        }
        n294 = case shown="True" "Add" {
          tunnel: w358 -> [_ w366]
          frame False {
          }
          frame True {
            n295 = local read "filename constr"() -> (w367:i32)
            n296 = Greater Or Equal?(x=w367, y=0) -> (x >= y?=w368:bool)
            n297 = case shown="True" w368 {
              tunnel: w367 -> [_ w378]
              tunnel: w366 -> [_ w381]
              frame False {
                n298 = call "CRYGet Error Message.vi"("Error No"=30, "Kind"="Auto Save") -> ("Message Sub 3"=w372:string, "Window Title"=w371:string)  [unwired: 4 in, 4 out]
                n299 = call "CRYMessage Dialog.vi"("Window Title"=w371, "YesNoCancel"=T7."OK", "Message Content"=w372) -> ()  [unwired: 7 in, 2 out]
              }
              frame True {
                n300 = local read "Template"() -> (w382:string)
                n301 = Index Array(array=w381, index=w378) -> (element=w387:string)
                n302 = Build Array (concatenate)("fn construction", w378) -> (w375:i32[])
                n303 = Empty String/Path?(string/path=w382) -> (empty?=w385:bool)
                n304 = Select(t="", s=w385, f=" ") -> (s? t:f=w383:string)
                n305 = property on="fn construction" class="Arr (strict)"("Val(Sgnl)"=w375) -> ()  [unwired: 2 in, 2 out]
                n306 = Concatenate Strings(w382, w383, w387) -> (w380:string)
                n307 = local read "Auto save"() -> (w377:T1)
                n308 = Bundle By Name(cluster=w377, "fn construction"=w375) -> (w376:T1)
                n309 = local write "Template"(w380) -> ()
                n310 = local write "Auto save"(w376) -> ()
              }
            }
          }
        }
      }
      event "Clear": Value Change {
        n311 = event-data() -> ()  [unwired: 7 out]
        n312 = case shown="True" "Clear" {
          frame False {
          }
          frame True {
            n313 = local write "Template"("") -> ()
            n314 = property on="fn construction" class="Arr (strict)"("Val(Sgnl)"=i32[] [] ("Value (Signaling)")) -> ()  [unwired: 2 in, 2 out]
          }
        }
      }
      event "Data List": Value Change {
        n315 = event-data() -> ("NewVal"=w395:i32[])  [unwired: 6 out]
        n316 = property on="Data List" class="LstBox (strict)"() -> ("Item Names"=w394:string[])  [unwired: 2 in, 2 out]
        n317 = for {
          tunnel: w395 -> [w398] mode=indexing
          tunnel: w394 -> [w397]
          tunnel: [w396] -> w393 mode=indexing
          n318 = Index Array(array=w397, index=w398) -> (element=w396:string)
        }
        n319 = local read "Auto save"() -> (w392:T1)
        n320 = Bundle By Name(cluster=w392, "Item Names"=w393) -> (w391:T1)
        n321 = local write "Auto save"(w391) -> ()
      }
      event "Autosave Folder Path:": Value Change {
        n322 = event-data() -> ("NewVal"=w401:path)  [unwired: 6 out]
        n323 = local read "Auto save"() -> (w400:T1)
        n324 = Bundle By Name(cluster=w400, "Autosave folder"=w401) -> (w399:T1)
        n325 = local write "Auto save"(w399) -> ()
      }
      event "File Name Mode2": Value Change {
        n326 = event-data() -> ("NewVal"=w405:u16)  [unwired: 6 out]
        n327 = case shown="1" w405 {
          tunnel: [T5."Enabled" ("Disabled") T5."Disabled and Grayed Out" ("Disabled")] -> w402
          frame 0, Default {
          }
          frame 1 {
          }
        }
        n328 = local read "Auto save"() -> (w404:T1)
        n329 = Bundle By Name(cluster=w404, "filename option"=w405) -> (w403:T1)
        n330 = local write "Auto save"(w403) -> ()
        n331 = property on="filename constr" class="LstBox (strict)"("DisabledEnum"=w402) -> ()  [unwired: 2 in, 2 out]
        n332 = property on="Template" class="Str"("DisabledEnum"=w402) -> ()  [unwired: 2 in, 2 out]
        n333 = property on="User defined" class="Str"("DisabledEnum"=w402) -> ()  [unwired: 2 in, 2 out]
        n334 = property on="Add" class="Bool"("DisabledEnum"=w402) -> ()  [unwired: 2 in, 2 out]
        n335 = property on="Clear" class="Bool"("DisabledEnum"=w402) -> ()  [unwired: 2 in, 2 out]
        n336 = property on="Selector" class="Ring (strict)"("DisabledEnum"=w402) -> ()  [unwired: 2 in, 2 out]
      }
      event "Layout Op": Value Change {
        n337 = event-data() -> ("NewVal"=w410:u16)  [unwired: 6 out]
        n338 = local read "Auto save"() -> (w409:T1)
        n339 = Bundle By Name(cluster=w409, "layout"=w410) -> (w408:T1)
        n340 = local write "Auto save"(w408) -> ()
      }
      event "Notation Op": Value Change {
        n341 = event-data() -> ("NewVal"=w413:u16)  [unwired: 6 out]
        n342 = local read "Auto save"() -> (w412:T1)
        n343 = Bundle By Name(cluster=w412, "notation"=w413) -> (w411:T1)
        n344 = local write "Auto save"(w411) -> ()
      }
      event "Notation Decimal": Value Change {
        n345 = event-data() -> ("NewVal"=w416:i32)  [unwired: 6 out]
        n346 = local read "Auto save"() -> (w415:T1)
        n347 = Bundle By Name(cluster=w415, "precision"=w416) -> (w414:T1)
        n348 = local write "Auto save"(w414) -> ()
      }
      event "Prompt for comment": Value Change {
        n349 = event-data() -> ("NewVal"=w419:bool)  [unwired: 6 out]
        n350 = local read "Auto save"() -> (w418:T1)
        n351 = Bundle By Name(cluster=w418, "prompt comment"=w419) -> (w417:T1)
        n352 = local write "Auto save"(w417) -> ()
      }
      event "Custom header": Value Change {
        n353 = event-data() -> ("NewVal"=w422:string)  [unwired: 6 out]
        n354 = local read "Auto save"() -> (w421:T1)
        n355 = Bundle By Name(cluster=w421, "custom header"=w422) -> (w420:T1)
        n356 = local write "Auto save"(w420) -> ()
      }
      event "Serial No.": Value Change {
        n357 = event-data() -> ("NewVal"=w425:bool)  [unwired: 6 out]
        n358 = local read "Auto save"() -> (w424:T1)
        n359 = Bundle By Name(cluster=w424, "serial no."=w425) -> (w423:T1)
        n360 = local write "Auto save"(w423) -> ()
      }
      event "User defined": Value Change {
        n361 = event-data() -> ("NewVal"=w428:string)  [unwired: 6 out]
        n362 = local read "Auto save"() -> (w427:T1)
        n363 = Bundle By Name(cluster=w427, "User defined"=w428) -> (w426:T1)
        n364 = local write "Auto save"(w426) -> ()
      }
      event "Character": Value Change {
        n365 = event-data() -> ("NewVal"=w431:string)  [unwired: 6 out]
        n366 = local read "Auto save"() -> (w430:T1)
        n367 = Bundle By Name(cluster=w430, "other delim"=w431) -> (w429:T1)
        n368 = local write "Auto save"(w429) -> ()
      }
      event "x": Value Change {
        n369 = event-data() -> ("NewVal"=w434:bool)  [unwired: 6 out]
        n370 = local read "Auto save"() -> (w433:T1)
        n371 = Bundle By Name(cluster=w433, "axes.x"=w434) -> (w432:T1)
        n372 = local write "Auto save"(w432) -> ()
      }
      event "y": Value Change {
        n373 = event-data() -> ("NewVal"=w437:bool)  [unwired: 6 out]
        n374 = local read "Auto save"() -> (w436:T1)
        n375 = Bundle By Name(cluster=w436, "axes.y"=w437) -> (w435:T1)
        n376 = local write "Auto save"(w435) -> ()
      }
      event "z": Value Change {
        n377 = event-data() -> ("NewVal"=w440:bool)  [unwired: 6 out]
        n378 = local read "Auto save"() -> (w439:T1)
        n379 = Bundle By Name(cluster=w439, "axes.z"=w440) -> (w438:T1)
        n380 = local write "Auto save"(w438) -> ()
      }
      event "Time": Value Change {
        n381 = event-data() -> ("NewVal"=w443:bool)  [unwired: 6 out]
        n382 = local read "Auto save"() -> (w442:T1)
        n383 = Bundle By Name(cluster=w442, "Time Stamp"=w443) -> (w441:T1)
        n384 = local write "Auto save"(w441) -> ()
      }
      event "Lot No.": Value Change {
        n385 = event-data() -> ("NewVal"=w446:bool)  [unwired: 6 out]
        n386 = local read "Auto save"() -> (w445:T1)
        n387 = Bundle By Name(cluster=w445, "Lot No."=w446) -> (w444:T1)
        n388 = local write "Auto save"(w444) -> ()
      }
      event "Operator": Value Change {
        n389 = event-data() -> ("NewVal"=w449:bool)  [unwired: 6 out]
        n390 = local read "Auto save"() -> (w448:T1)
        n391 = Bundle By Name(cluster=w448, "Operator"=w449) -> (w447:T1)
        n392 = local write "Auto save"(w447) -> ()
      }
      event "fn construction": Value Change {
        w455 = T5."Disabled and Grayed Out" ("Disabled")
        w465 = T5."Enabled" ("Disabled")
        w467 = ""
        n393 = event-data() -> ("NewVal"=w453:i32[])  [unwired: 6 out]
        n394 = global read "CRYMainGlobal.vi" "Language"() -> (w451:T6)
        n395 = case shown="\"Chinese\"" w451 {
          tunnel: [string[] ["<\u0000s\u0000e\u0000q\u0000>\u0000", "<\u0000l\u0000o\u0000t\u0000>\u0000", "<\u0000u\u0000s\u0000e\u0000r\u0000>\u0000", "<\u0000s\u0000n\u0000>\u0000", "<\u0000d\u0000a\u0000t\u0000e\u0000>\u0000", "<\u0000t\u0000i\u0000m\u0000e\u0000>\u0000", "<\u0000d\u0000 \u0000o\u0000r\u0000 \u0000r\u0000>\u0000", "<\u0000c\u0000l\u0000v\u0000a\u0000l\u0000>\u0000", "<\u0000o\u0000p\u0000e\u0000r\u0000>\u0000"] string[] ["<\u0000^\u0017R\rTðy>\u0000", "<\u0000ÁT\rT>\u0000", "<\u0000ꁚ[IN>\u0000", "<\u0000^\u0017R÷S>\u0000", "<\u0000åe\u001fg>\u0000", "<\u0000öeô•>\u0000", "<\u0000penc\u0016bÓ~œg\u0016bâl>\u0000", "<\u0000òf¿~“^<P>\u0000", "<\u0000Íd\\OXT>\u0000"]] -> w452
          frame "English", Default {
          }
          frame "Chinese" {
          }
        }
        n396 = Search 1D Array(1D array=w453, element=u16 2) -> (index of element=w458:i32)  [unwired: 1 in]
        n397 = Search 1D Array(1D array=w453, element=u16 7) -> (index of element=w461:i32)  [unwired: 1 in]
        n398 = Equal?(x=w461, y=-1) -> (x = y?=w464:bool)
        n399 = Equal?(x=w458, y=-1) -> (x = y?=w463:bool)
        n400 = Select(t=w455, s=w463, f=w465) -> (s? t:f=w456:T5)
        n401 = Select(t=w455, s=w464, f=w465) -> (s? t:f=w454:T5)
        n402 = for {
          tunnel: [w471] -> w450 mode=indexing
          tunnel: w452 -> [w470] mode=indexing
          n403 = call "CRYConvert Unicode to ASCII.vi"("Unicode"=w470) -> ("ASCII"=w471:string)  [unwired: 4 in]
        }
        n404 = property on="User defined" class="Str"("DisabledEnum"=w456) -> ()  [unwired: 2 in, 2 out]
        n405 = property on="Value" class="Ring (strict)"("DisabledEnum"=w454) -> ()  [unwired: 2 in, 2 out]
        n406 = property on="Axis" class="Slide (strict)"("DisabledEnum"=w454) -> ()  [unwired: 2 in, 2 out]
        n407 = local read "Auto save"() -> (w469:T1)
        n408 = property on="single val" class="Str"("DisabledEnum"=w454) -> ()  [unwired: 2 in, 2 out]
        n409 = for {
          shift-right: [w474] -> w466
          shift-left: w467 -> [w478]
          tunnel: w467 -> [w479]
          tunnel: w453 -> [w477] mode=indexing
          tunnel: w450 -> [w476]
          n410 = Index Array(array=w476, index=w477) -> (element=w475:string)
          n411 = Empty String/Path?(string/path=w478) -> (empty?=w482:bool)
          n412 = Select(t=w479, s=w482, f=" ") -> (s? t:f=w480:string)
          n413 = Concatenate Strings(w478, w480, w475) -> (w474:string)
        }
        n414 = Bundle By Name(cluster=w469, "fn construction"=w453) -> (w468:T1)
        n415 = property on="Format Value" class="Bool"("DisabledEnum"=w454) -> ()  [unwired: 2 in, 2 out]
        n416 = local write "Auto save"(w468) -> ()
        n417 = local write "Template"(w466) -> ()
      }
      event "Help": Value Change {
        n418 = event-data() -> ("NewVal"=w485:string)  [unwired: 6 out]
        n419 = local read "Auto save"() -> (w484:T1)
        n420 = Bundle By Name(cluster=w484, "Help"=w485) -> (w483:T1)
        n421 = local write "Auto save"(w483) -> ()
      }
      event "Value": Value Change {
        n422 = event-data() -> ("NewVal"=w489:u16)  [unwired: 6 out]
        n423 = property on="Value" class="Ring (strict)"() -> ("Strings []"=w487:string[])  [unwired: 2 in, 2 out]
        n424 = local read "Axis"() -> (w486:u16)
        n425 = Index Array(array=w487, index=w489) -> (element=w488:string)
        n426 = local read "Auto save"() -> (w491:T1)
        n427 = Bundle By Name(cluster=w491, "Value Name"=w488) -> (w490:T1)
        n428 = property on="Axis" class="Slide (strict)"("Val(Sgnl)"=w486) -> ()  [unwired: 2 in, 2 out]
        n429 = local write "Auto save"(w490) -> ()
      }
      event "Axis": Value Change {
        n430 = event-data() -> ("NewVal"=w498:u16)  [unwired: 6 out]
        n431 = property on="Value" class="Ring (strict)"() -> ("Strings []"=w496:string[])  [unwired: 2 in, 2 out]
        n432 = local read "Value"() -> (w503:u16)
        n433 = local read "Auto save"() -> (w495:T1)
        n434 = Index Array(array=w496, index=w503) -> (element=w497:string)
        n435 = Bundle By Name(cluster=w495, "Axis"=w498) -> (w504:T1)
        n436 = local write "Auto save"(w504) -> ()
        n437 = call "CRYGet Curve Library One Data .vi"("Data Name"=w497, "Type"=enum16{"Curves", "Values", "Results", "WFM"}."Values") -> ("Value"=w501:T9)  [unwired: 3 in, 6 out]
        n438 = Unbundle By Name(w501) -> ("Curve"=w500:cluster{"x":dbl, "y":dbl, "z":dbl}[])
        n439 = Unbundle By Name(w495) -> ("format string.Lin Format String out"=w494:string)
        n440 = Index Array(array=w500) -> (element=w499:cluster{"x":dbl, "y":dbl, "z":dbl})  [unwired: 1 in]
        n441 = case shown="0, Default" w498 {
          tunnel: w499 -> [w506 w508 w510]
          tunnel: [w505 w507 w509] -> w493
          frame 0, Default {
            n442 = Unbundle By Name(w506) -> ("x"=w505:dbl)
          }
          frame 1 {
            n443 = Unbundle By Name(w508) -> ("y"=w507:dbl)
          }
          frame 2 {
            n444 = Unbundle By Name(w510) -> ("z"=w509:dbl)
          }
        }
        n445 = call "CRYGet Formated String Value.vi"("Value"=w493, "Flattened Format String"=w494) -> ("Unflattened Format string"=w492:string)  [unwired: 9 in]
        n446 = local write "single val"(w492) -> ()
      }
      event "Format Value": Value Change {
        n447 = event-data() -> ()  [unwired: 7 out]
        n448 = case shown="True" "Format Value" {
          frame False {
          }
          frame True {
            n449 = flat-sequence {
              frame #0 {
                n450 = local read "Auto save"() -> (w515:T1)
                n451 = Unbundle By Name(w515) -> ("format string.Lin Format String out"=w513:string)
                n452 = call "CRYRead format string.vi"("Format string"=w513) -> ("Notation"=w516:u16, "Digits"=w517:u16, "Precision"=w518:u16, "Hide Traling Zeros"=w519:bool)  [unwired: 7 in]
                n453 = call "CRYNumber Format.vi"("Notation"=w516, "Digits"=w517, "Precision"=w518, "Hide Trailing Zeros"=w519) -> ("Format string"=w512:string)  [unwired: 7 in]
                n454 = Bundle By Name(cluster=w515, "format string.Lin Format String out"=w512) -> (w514:T1)
                n455 = local write "Auto save"(w514) -> ()
              }
              frame #1 {
                n456 = property on="Axis" class="Slide (strict)"() -> ("Value"=w520:u16)  [unwired: 2 in, 2 out]
                n457 = property on="Axis" class="Slide (strict)"("Val(Sgnl)"=w520) -> ()  [unwired: 2 in, 2 out]
              }
            }
          }
        }
      }
      event "Main Tab": Value Change {
        n458 = event-data() -> ("NewVal"=w523:enum32{"Setting", "Help"})  [unwired: 6 out]
        n459 = local read "Auto save"() -> (w522:T1)
        n460 = Bundle By Name(cluster=w522, "Tab Value"=w523) -> (w521:T1)
        n461 = local write "Auto save"(w521) -> ()
      }
    }
    n462 = global read "CRYMain Sub Window Global.vi" "gStop"() -> (w39:bool)
    n463 = Or(x=w39, y="stop") -> (x .or. y?=w38:bool)
    n464 = Bundle("Apply"="Apply", "Load Test"="Load Test", "OK"="OK", "Cancel"="Cancel") -> (w43:T14)  [unwired: 1 out]
    n465 = Cluster To Array(cluster=w43) -> (array=w42:bool[])
    n466 = Search 1D Array(1D array=w42, element=TRUE) -> (index of element=w40:i32)  [unwired: 1 out]
    n467 = case shown="1" w40 {
      frame Default {
      }
      frame 0 {
        n468 = global read "CRYMainGlobal.vi" "Access Level"() -> (w45:enum16{"Engineer", "Technician", "Operator"})
        n469 = case shown="\"Operator\", Default" w45 {
          frame "Engineer" {
            n470 = flat-sequence {
              tunnel: [w47] -> w46
              tunnel: w46 -> [w52]
              frame #0 {
                n471 = call "CRYGet Current TS Steps.vi"() -> ("SelectStepNumber in Tree"=w48:i32, "Steps"=w49:T4[])  [unwired: 1 in, 9 out]
                n472 = Index Array(array=w49, index=w48) -> (element=w47:T4)
              }
              frame #1 {
                n473 = local read "Auto save"() -> (w50:T1)
                n474 = call "CRYFlatten Auto Save.vi"("Auto Save"=w50) -> ("Auto Save flattened"=w54:string)  [unwired: 10 in]
                n475 = Bundle By Name(cluster=w52, "Seq setup flattened"=w54) -> (w53:T4)
                n476 = Unbundle By Name(w52) -> ("StepName"=w51:string)
                n477 = call "CRYAuto Save.vi"("Setup in"=w53, "Step name"=w51) -> ()  [unwired: 9 in, 5 out]
              }
            }
          }
          frame "Operator", Default {
            n478 = call "CRYGet Error Message.vi"("Kind"="Step Setup") -> ("Window Title"=w56:string)  [unwired: 5 in, 5 out]
            n479 = call "CRYGet Access Level Message.vi"() -> ("Multibyte string"=w58:string)  [unwired: 11 in]
            n480 = call "CRYMessage Dialog.vi"("Window Title"=w56, "YesNoCancel"=T7."OK", "Message Content"=w58) -> ()  [unwired: 7 in, 2 out]
          }
        }
      }
      frame 1 {
        n481 = flat-sequence {
          frame #0 {
            n482 = local read "Auto save"() -> (w78:T1)
            n483 = Unbundle By Name(w78) -> ("User Default"=w59:bool, "save"=w99:enum16{"Data", "Results", "Waveforms"}, "Item Names"=→"Data Names":string[], "Autosave folder"=w98:path, "data format"=w76:u16, "filename option"=w70:enum16{"auto", "prompt"}, "fn construction"=w80:i32[], "layout"=w97:enum16{"rows", "columns"}, "notation"=w96:enum16{"sci", "float"}, "precision"=w95:i32, "prompt comment"=w94:bool, "header"=w93:enum16{"none", "standard", "custom"}, "custom header"=w92:string, "serial no."=w91:bool, "User defined"=w90:string, "delimiter"=w89:enum16{"tab", "comma", "space", "other"}, "other delim"=w88:string, "axes"=w84:cluster{"x":bool, "y":bool, "z":bool}, "Time Stamp"=w85:bool, "Lot No."=w87:bool, "Operator"=w86:bool, "New or Append"=w77:u16, "Help"=w74:string, "Tab Value"=w79:enum32{"Setting", "Help"}, "Excel Template"=w73:string, "Selector"=w72:i32, "Axis"=w65:u16, "Value Name"=w66:string, "DBPath"=w60:path)
            n484 = call "CRYGet Curve Library Data Name.vi"("sAction"="GetNameByType", "Type"=enum16{"Curves", "Values", "Results", "WFM"}."Values") -> ("sNames"=w67:string[])  [unwired: 6 in, 3 out]
            n485 = Search 1D Array(1D array=w67, element=w66) -> (index of element=w62:i32)  [unwired: 1 in]
            n486 = local write "DBPath"(w60) -> ()
            n487 = String To Path(string=w73) -> (path=w71:path)
            n488 = Less Than 0?(x=w62) -> (x < 0?=w64:bool)
            n489 = Select(t=0, s=w64, f=w62) -> (s? t:f=w61:i32)
            n490 = flat-sequence {
              tunnel: w61 -> [w100]
              tunnel: w65 -> [w101]
              frame #0 {
                n491 = local write "Value"(w100) -> ()
              }
              frame #1 {
                n492 = property on="Axis" class="Slide (strict)"("Val(Sgnl)"=w101) -> ()  [unwired: 2 in, 2 out]
              }
            }
            n493 = local write "Prompt for comment"(w94) -> ()
            n494 = local write "Notation Decimal"(w95) -> ()
            n495 = local write "File Name Mode1"(w77) -> ()
            n496 = local write "Notation Op"(w96) -> ()
            n497 = local write "Custom header"(w92) -> ()
            n498 = local write "Delimiter"(w89) -> ()
            n499 = property on="Save Op" class="Slide (strict)"("Val(Sgnl)"=w99) -> ()  [unwired: 2 in, 2 out]
            n500 = local write "Autosave Folder Path:"(w98) -> ()
            n501 = local write "Format Op"(w76) -> ()
            n502 = property on="fn construction" class="Arr (strict)"("Val(Sgnl)"=w80) -> ()  [unwired: 2 in, 2 out]
            n503 = local write "User defined"(w90) -> ()
            n504 = local write "Layout Op"(w97) -> ()
            n505 = local write "Header Op"(w93) -> ()
            n506 = local write "Serial No."(w91) -> ()
            n507 = local write "Time"(w85) -> ()
            n508 = local write "Lot No."(w87) -> ()
            n509 = property on="Main Tab" class="TabCtl (strict)"("Value"=w79) -> ()  [unwired: 2 in, 2 out]
            n510 = local write "Character"(w88) -> ()
            n511 = local write "Operator"(w86) -> ()
            n512 = local write "Help"(w74) -> ()
            n513 = local write "Excel Path"(w71) -> ()
            n514 = local write "Selector"(w72) -> ()
            n515 = property on="User Default" class="Bool (strict)"("Val(Sgnl)"=w59) -> ()  [unwired: 2 in, 2 out]
            n516 = property on="File Name Mode2" class="Slide (strict)"("Val(Sgnl)"=w70) -> ()  [unwired: 2 in, 2 out]
            n517 = Unbundle By Name(w84) -> ("x"=w83:bool, "y"=w82:bool, "z"=w81:bool)
            n518 = local write "y"(w82) -> ()
            n519 = local write "z"(w81) -> ()
            n520 = local write "x"(w83) -> ()
          }
          frame #1 {
            n521 = control-ref of="Board Tab"() -> (w103:refnum<vi>)
            n522 = control-ref of="This VI"() -> (w102:refnum<vi>)
            n523 = call "CRYAlign Steps VI Center.vi"("Tab2"=w103, "Input/Output"=TRUE ("Preview"), "VIRef"=w102) -> ()  [unwired: 1 in, 8 out]
          }
          frame #2 {
            n524 = local write "Load Test"(FALSE ("Load Test")) -> ()
            n525 = property on="Board Tab" class="TabCtl (strict)"("Visible"=TRUE) -> ()  [unwired: 2 in, 2 out]
          }
        }
      }
      frame 2 {
        n526 = global read "CRYMainGlobal.vi" "Access Level"() -> (w107:enum16{"Engineer", "Technician", "Operator"})
        n527 = local write "OK"(FALSE ("OK")) -> ()
        n528 = local write "stop"(TRUE ("stop")) -> ()
        n529 = case shown="\"Technician\", Default" w107 {
          frame "Engineer" {
            n530 = local read "Auto save"() -> (w111:T1)
            n531 = local read "Proper VI No"() -> (w113:i32)
            n532 = call "CRYFlatten Auto Save.vi"("Auto Save"=w111) -> ("Auto Save flattened"=w110:string)  [unwired: 10 in]
            n533 = call "CRYPreUpdate Sequence.vi"("EventName"="SequenceUpdate", "Proper VI No"=w113, "Project View Step Name Identifier Arg1"="", "Step flattened Arg2"=w110, "AllChangeFlg"=TRUE ("Name/Identifier")) -> ()  [unwired: 11 in]
          }
          frame "Technician", Default {
            n534 = call "CRYGet Error Message.vi"("Kind"="Step Setup") -> ("Window Title"=w118:string)  [unwired: 5 in, 5 out]
            n535 = call "CRYGet Access Level Message.vi"("sAction"="OK") -> ("Multibyte string"=w120:string)  [unwired: 10 in]
            n536 = call "CRYMessage Dialog.vi"("Window Title"=w118, "YesNoCancel"=T7."OK", "Message Content"=w120) -> ()  [unwired: 7 in, 2 out]
          }
        }
      }
      frame 3 {
        n537 = local write "Cancel"(FALSE ("Cancel")) -> ()
        n538 = local write "stop"(TRUE ("stop")) -> ()
      }
    }
  }
  n539 = flat-sequence {
    tunnel: w2 -> [_]
    frame #0 {
      n540 = control-ref of="This VI"() -> (w524:refnum<vi>)
      n541 = call "CRYWork Before Step Close.vi"("StepVI Ref"=w524) -> ()  [unwired: 11 in]
    }
    frame #1 {
      n542 = local write "EndFlag"(TRUE ("EndFlag")) -> ()
    }
  }
